vi "Serial_NumberCheck.vi"(10 "Serial Number In":string) -> (1 "Serial Number":bool, 3 "Serial number out":string)   [LabVIEW 2019]
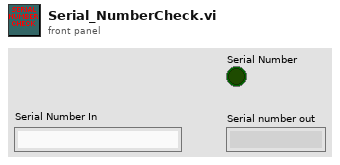
[diagram p1: front panel]
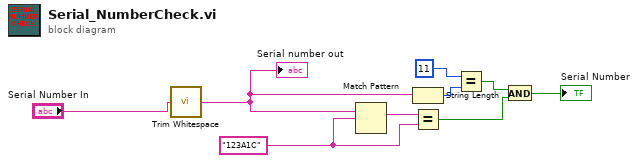
[diagram p0: block diagram]
diagram:
  w8 = "123A1C"
  n1 = call <vilib>:"Trim Whitespace.vi"("string"="Serial Number In") -> ("trimmed string"=w1:string)  [unwired: 1 in]
  "Serial number out" <- w1
  n2 = Match Pattern(string=w1, regular expression=w8) -> (match substring=w9:string)  [unwired: 1 in, 3 out]
  n3 = String Length(string=w1) -> (length=w7:i32)
  n4 = Equal?(x=w9, y=w8) -> (x = y?=w4:bool)
  n5 = Equal?(x=11, y=w7) -> (x = y?=w5:bool)
  n6 = And(x=w5, y=w4) -> (x .and. y?=→"Serial Number":bool)
